vi "CalcWrist.vi"(5 "Teleop Local Data Out in":T1 {"Vision"."Theta_Y" format="%.1f"; "Vision"."Theta_X" format="%.1f"; "Potentio" format="%.1f"; "Drive_Enc_R" format="%.1f"; "Drive_Enc_L" format="%.1f"; "Gyro_Angle" format="%.1f"; "Encoder_Lift" format="%.1f"; "Motor_Lift" format="%.3f"; "Motor_Intake" format="%.3f"; "Drive_Twist" format="%.3f"; "Drive_Forward" format="%.3f"}, 9 "error in (no error)":errorcluster) -> (6 "Teleop Local Data Out out":T1 {"Vision"."Theta_Y" format="%.1f"; "Vision"."Theta_X" format="%.1f"; "Potentio" format="%.1f"; "Drive_Enc_R" format="%.1f"; "Drive_Enc_L" format="%.1f"; "Gyro_Angle" format="%.1f"; "Encoder_Lift" format="%.1f"; "Motor_Lift" format="%.3f"; "Motor_Intake" format="%.3f"; "Drive_Twist" format="%.3f"; "Drive_Forward" format="%.3f"}, 10 "error out":errorcluster)   [LabVIEW 2018]
uses:
  Typedefs/typedef_cluster_TeleOp_Local_Data.ctl
  Typedefs/typedef_cluster_Joystick.ctl
  Typedefs/typedef_cluster_Vision.ctl
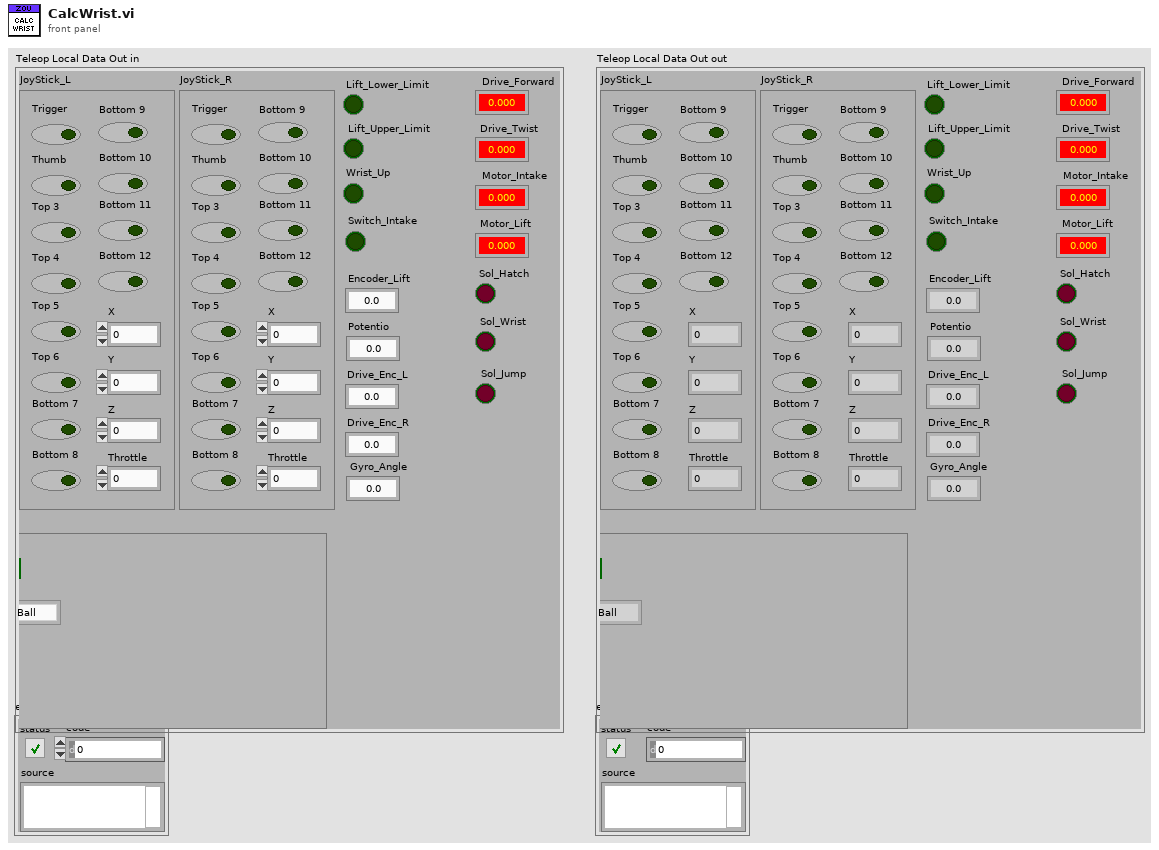
[diagram p1: front panel]
types:
  T1 = typedef "typedef_cluster_TeleOp_Local_Data.ctl" = cluster{"Lift_Lower_Limit":bool, "Wrist_Up":bool, "Switch_Intake":bool, "Encoder_Lift":dbl, "Sol_Wrist":bool, "Motor_Intake":dbl, "Motor_Lift":dbl, "Drive_Forward":dbl, "Drive_Twist":dbl, "Sol_Hatch":bool, "Gyro_Angle":dbl, "Drive_Enc_L":dbl, "Drive_Enc_R":dbl, "JoyStick_L":T2, "JoyStick_R":T2, "Potentio":dbl, "Vision":T3, "Lift_Upper_Limit":bool, "Sol_Jump":bool}
  T2 = typedef "typedef_cluster_Joystick.ctl" = cluster{"X":dbl, "Y":dbl, "Z":dbl, "Throttle":dbl, "Trigger":bool, "Thumb":bool, "Top 3":bool, "Top 4":bool, "Top 5":bool, "Top 6":bool, "Bottom 7":bool, "Bottom 8":bool, "Bottom 9":bool, "Bottom 10":bool, "Bottom 11":bool, "Bottom 12":bool}
  T3 = typedef "typedef_cluster_Vision.ctl" = cluster{"Theta_X":dbl, "Theta_Y":dbl, "Has_Target":bool, "Seek_Ball":bool, "Pipeline":enum16{"Ball", "Dual_Target", "Single_Target"}}
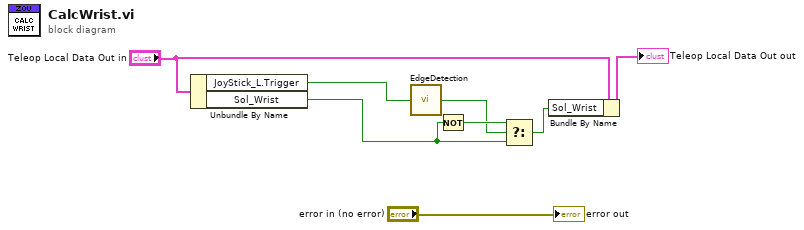
[diagram p0: block diagram]
diagram:
  n1 = Unbundle By Name("Teleop Local Data Out in") -> ("JoyStick_L.Trigger"=w2:bool, "Sol_Wrist"=w1:bool)
  n2 = call "EdgeDetection.vi"("Boolean"=w2) -> ("Boolean 2"=w4:bool)  [unwired: 14 in]
  n3 = Not(x=w1) -> (.not. x?=w5:bool)
  n4 = Select(t=w5, s=w4, f=w1) -> (s? t:f=w3:bool)
  n5 = Bundle By Name(cluster="Teleop Local Data Out in", "Sol_Wrist"=w3) -> (→"Teleop Local Data Out out":T1)
  "error out" <- "error in (no error)"
